vi "Add Subordinate.vi"(8 "error in (no error)":errorcluster, 10 "Subordinate":T1, 11 "Managed Actor in":refnum<class "Managed Actor.lvclass">) -> (0 "error out":errorcluster, 3 "Managed Actor out":refnum<class "Managed Actor.lvclass">)   [LabVIEW 2023, in "Engine.lvlib" / "Managed Actor.lvlib" / "Managed Actor.lvclass"]
doc: "<b>Add Subordinate</b> inserts a subordinate record into the map for management."
uses:
  Library/Managed Actor.lvclass
  Custom Controls/Subordinate.ctl
  builds/Framework/Actor Framework.lvlibp/1abvi3w/vi.lib/ActorFramework/Message Enqueuer/Message Enqueuer.lvclass
  Library/Managed Actor.lvclass/Managed Actor.ctl
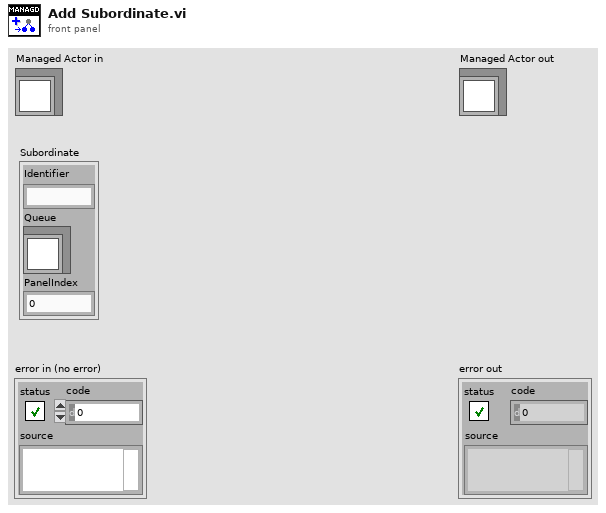
[diagram p1: front panel]
types:
  T1 = typedef "Engine.lvlib/Managed Actor.lvlib/Managed Actor.lvclass/Subordinate.ctl" = cluster{"Identifier":string, "Queue":refnum<class "Message Enqueuer.lvclass">, "PanelIndex":i32}
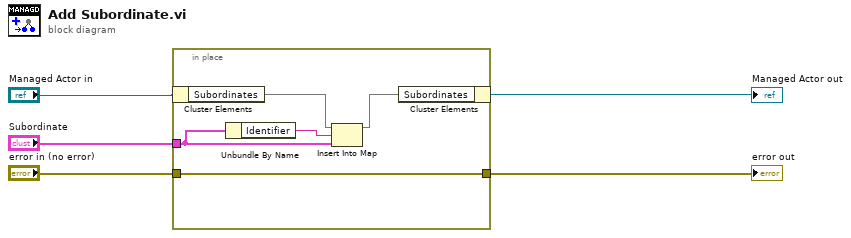
[diagram p0: block diagram]
diagram:
  n1 = in-place {
    in-place-border: "error in (no error)" -> [w6]
    in-place-border: "Subordinate" -> [w8]
    in-place-border: [w6] -> w1
    n2 = in-place-cluster #1("Managed Actor in") -> ("Subordinates"=w10:map{string, T1})
    n3 = Unbundle By Name(w8) -> ("Identifier"=w7:string)
    n4 = Insert Into Map(map in=w10, key=w7, value=w8) -> (map out=w9:map{string, T1})  [unwired: 2 out]
    n5 = in-place-cluster #1("Subordinates"=w9) -> (→"Managed Actor out":refnum<class "Managed Actor.lvclass">)
  }
  "error out" <- w1
